vi "APC_isProblem.vi"(8 "error in (no error)":errorcluster) -> (0 "error out":errorcluster, 3 "PowerProblem?":bool)   [LabVIEW 2018]
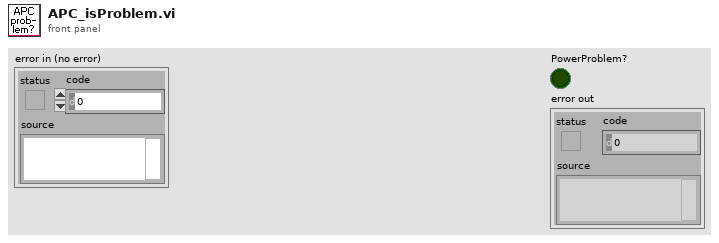
[diagram p1: front panel]
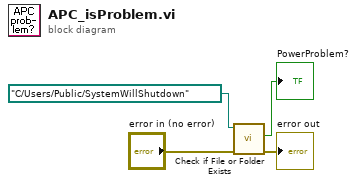
[diagram p0: block diagram]
diagram:
  n1 = call <vilib>:"Check if File or Folder Exists.vi"("error in (no error)"="error in (no error)", "path"=path "C:/Users/Public/SystemWillShutdown" ("path (use dialog)")) -> ("error out"=→"error out":errorcluster, "file or folder exists?"=→"PowerProblem?":bool)  [unwired: 7 in, 1 out]
